vi "SDCP SMF Transmitter and Receiver - Obtain Plot Points from Trace File.vi"(4 "Stop file index":u16, 6 "error in (no error)":errorcluster, 7 "Trace File Path":path=path "E:/Projects/System Diagnostics and Control Protocol/SDCP_LabVIEW/temp/Trace Files/21 Apr 2024 20-17.csv", 8 "Start file index":u16, 10 "Parameter file path":path=path "E:/Projects/System Diagnostics and Control Protocol/SDCP_LabVIEW/Parameter Files/Motion_Processing.param") -> (0 "error out":errorcluster, 2 "Parameter names":string[](array[string]), 3 "Plot details":T1(array[cluster]))   [LabVIEW 2020]
panel:
  out "File counter":i32
  out "Frame Counter":u16
  in  "Parameter Length":i32=1
  in  "Parameter Start Index":i32=26
  out "XY Graph":T2(graph)
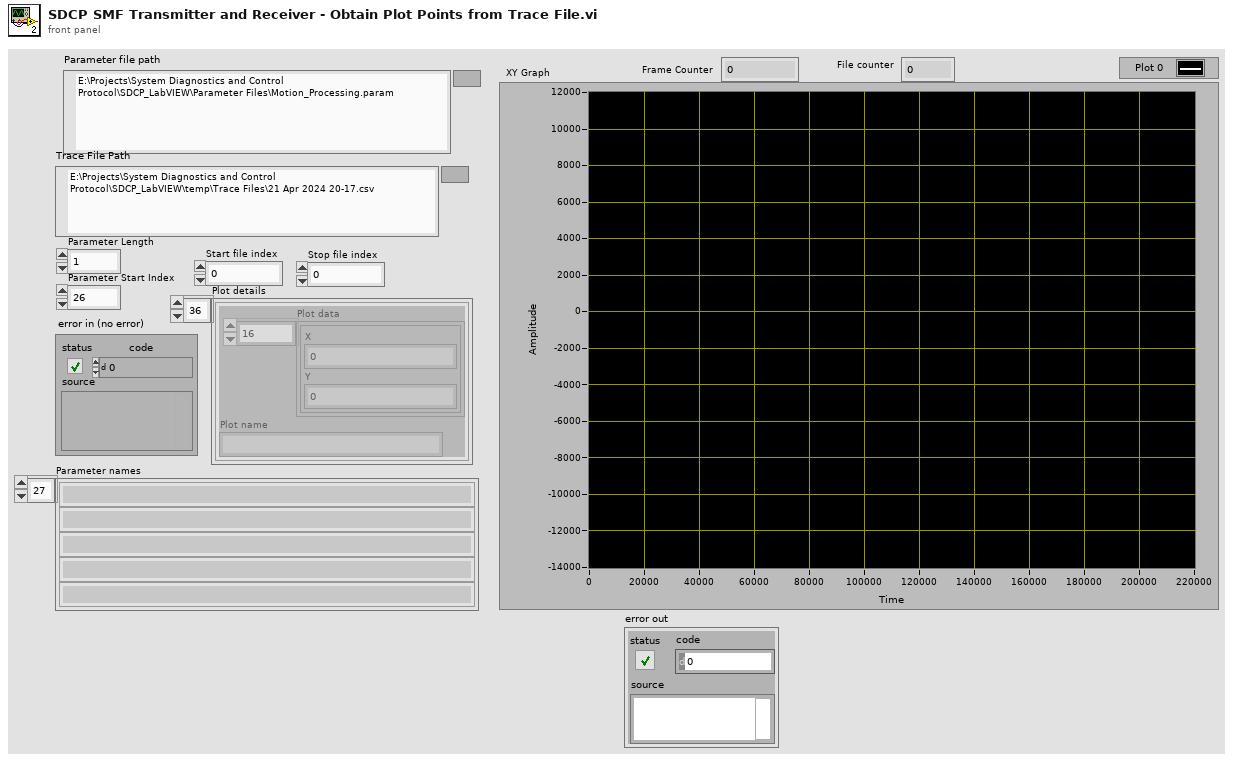
[diagram p1: front panel]
types:
  T1 = cluster{"Plot data":cluster{"X":dbl, "Y":dbl}[], "Plot name":string}[]
  T2 = cluster{"Plot data":cluster{"X":dbl, "Y":dbl}[]}[]
  T3 = cluster{"Plot data":cluster{"X":dbl, "Y":dbl}[], "Plot name":string}
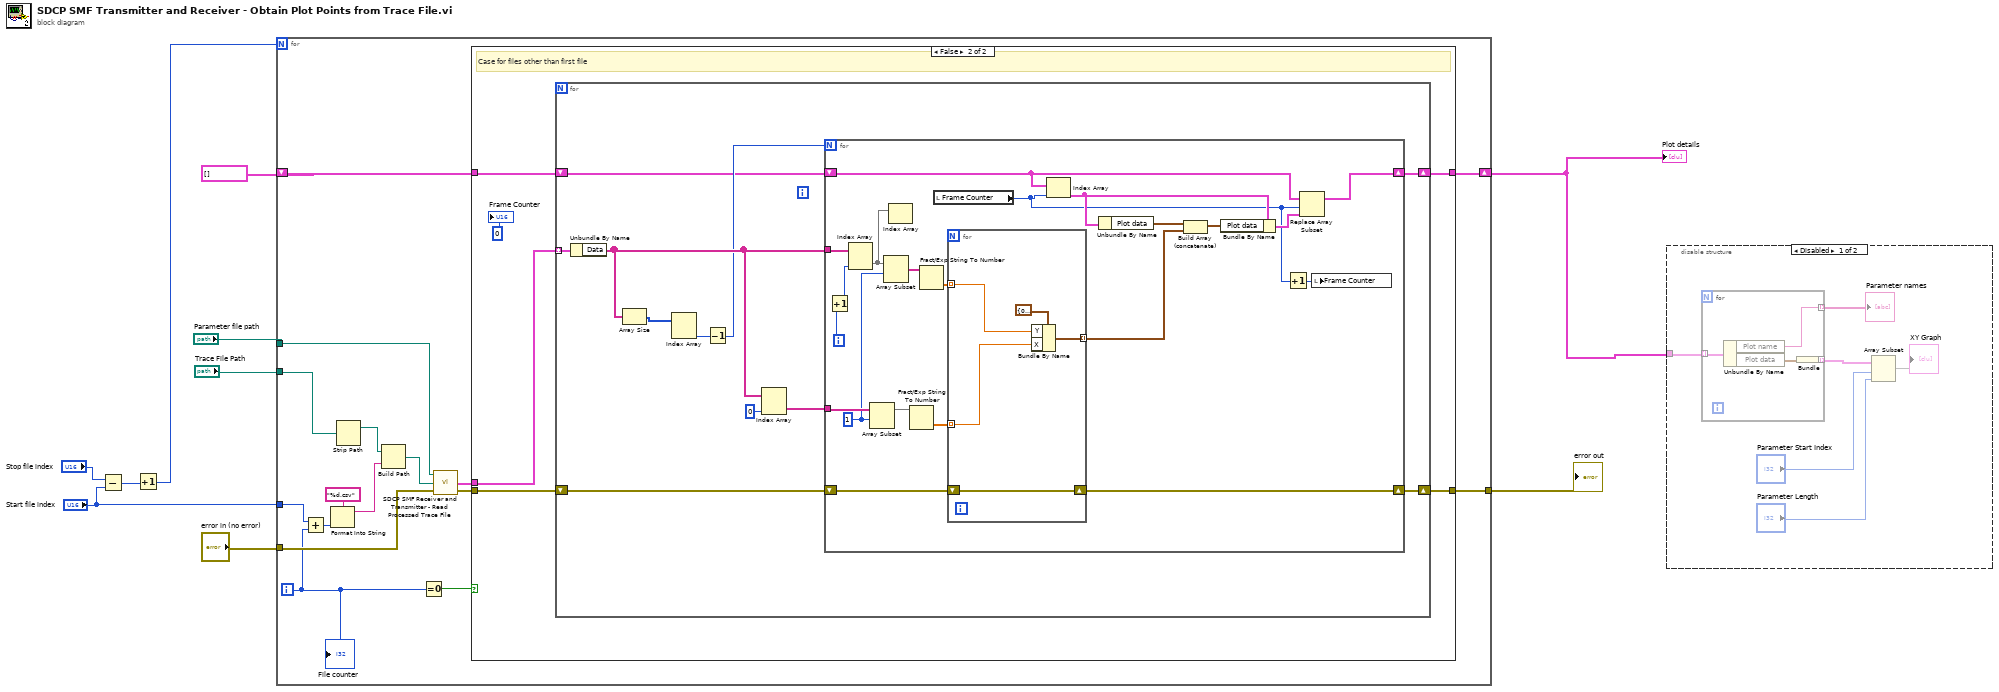
[diagram p0: block diagram]
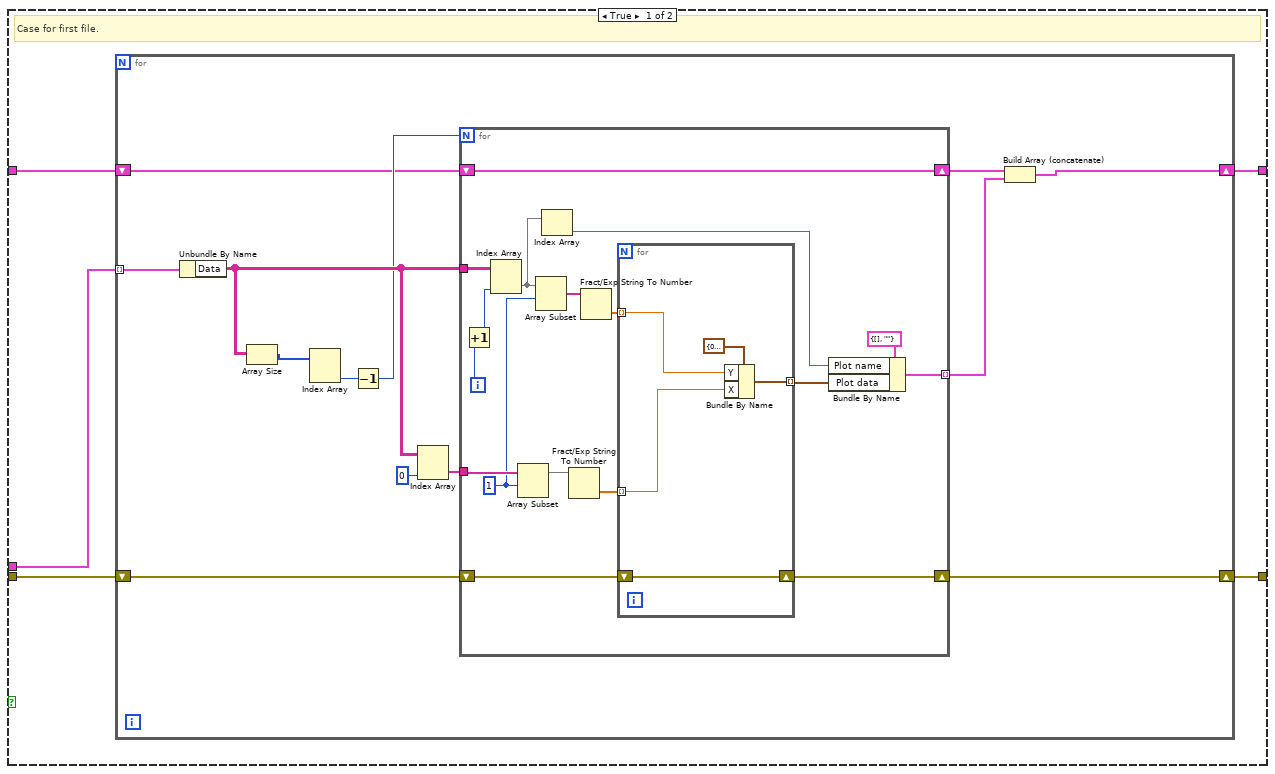
[diagram p3: hidden frame]
diagram:
  n1 = Subtract(x="Stop file index", y="Start file index") -> (x-y=w2:u16)
  n2 = Increment(x=w2) -> (x+1=w1:u16)
  n3 = for {
    N: w1 -> [_]
    tunnel: "Parameter file path" -> [w26]
    tunnel: "Trace File Path" -> [w20]
    tunnel: "error in (no error)" -> [w25]
    shift-right: [w21] -> w6
    shift-left: T1 [] -> [w22]
    tunnel: [w15] -> w5
    tunnel: "Start file index" -> [w11]
    i -> [w12]
    n4 = Add(x=w11, y=w12) -> (x+y=w13:i32)
    n5 = Format Into String(format string="%d.csv", w13) -> (resulting string=w16:string)  [unwired: 2 in, 1 out]
    n6 = Strip Path(path=w20) -> (stripped path=w19:path)  [unwired: 1 out]
    n7 = Build Path(base path=w19, name or relative path=w16) -> (appended path=w18:path)
    n8 = Equal To 0?(x=w12) -> (x = 0?=w14:bool)
    n9 = call "SDCP SMF Receiver and Transmitter - Read Processed Trace File.vi"("error in (no error)"=w25, "Trace File Path"=w18, "Parameter file path"=w26) -> ("error out"=w24:errorcluster, "Framewise output"=w23:cluster{"Data":string[][]}[])  [unwired: 1 out]
    n10 = case shown="False" w14 {
      tunnel: w24 -> [w31 w72]
      tunnel: w23 -> [w30 w71]
      tunnel: w22 -> [w29 w70]
      tunnel: [w28 w69] -> w21
      tunnel: [w27 w68] -> w15
      frame True {
        # "Case for first file."
        n11 = for {
          shift-right: [w37] -> w27
          shift-left: w31 -> [w41]
          tunnel: w30 -> [w44] mode=indexing
          shift-right: [w33] -> w28
          shift-left: w29 -> [w36]
          n12 = Unbundle By Name(w44) -> ("Data"=w40:string[][])
          n13 = Array Size(array=w40) -> (size(s)=w43:i32[])
          n14 = Index Array(array=w43) -> (element #2=w42:i32)  [unwired: 2 in, 1 out]
          n15 = Decrement(x=w42) -> (x-1=w39:i32)
          n16 = Index Array(array=w40, index (col)=0 ("disabled index (col)")) -> (element=w38:string[])  [unwired: 1 in]
          n17 = for {
            N: w39 -> [_]
            shift-right: [w46] -> w37
            shift-left: w41 -> [w47]
            tunnel: w40 -> [w61]
            tunnel: w38 -> [w55]
            tunnel: [w49] -> w34 mode=indexing
            shift-right: [w48] -> w35
            shift-left: w36 -> [w48]
            i -> [w60]
            w52 = 1 ("index")
            n18 = Increment(x=w60) -> (x+1=w45:i32)
            n19 = Index Array(array=w61, index (col)=w45) -> (element=w51:string[])  [unwired: 1 in]
            n20 = Array Subset(array=w55, index=w52) -> (w54:string[])  [unwired: 1 in]
            n21 = Array Subset(array=w51, index=w52) -> (w53:string[])  [unwired: 1 in]
            n22 = Index Array(array=w51) -> (element=w50:string)  [unwired: 1 in]
            n23 = Fract/Exp String To Number(string=w54) -> (number=w58:dbl[])  [unwired: 3 in, 1 out]
            n24 = Fract/Exp String To Number(string=w53) -> (number=w59:dbl[])  [unwired: 3 in, 1 out]
            n25 = for {
              tunnel: w59 -> [w64] mode=indexing
              tunnel: w58 -> [w65] mode=indexing
              tunnel: [w63] -> w56 mode=indexing
              shift-right: [w62] -> w46
              shift-left: w47 -> [w62]
              n26 = Bundle By Name(cluster=cluster{"X":dbl, "Y":dbl} {"X"=0.0, "Y"=0.0}, "Y"=w64, "X"=w65) -> (w63:cluster{"X":dbl, "Y":dbl})
            }
            n27 = Bundle By Name(cluster=T3 {"Plot data"=[], "Plot name"=""}, "Plot name"=w50, "Plot data"=w56) -> (w49:T3)
          }
          n28 = Build Array (concatenate)(w35, w34) -> (w33:T1)
        }
      }
      frame False {
        # "Case for files other than first file"
        n29 = for {
          shift-right: [w76] -> w68
          shift-left: w72 -> [w80]
          tunnel: w71 -> [w83] mode=indexing
          shift-right: [w74] -> w69
          shift-left: w70 -> [w75]
          n30 = Unbundle By Name(w83) -> ("Data"=w79:string[][])
          n31 = Array Size(array=w79) -> (size(s)=w82:i32[])
          n32 = Index Array(array=w82) -> (element #2=w81:i32)  [unwired: 2 in, 1 out]
          n33 = Decrement(x=w81) -> (x-1=w78:i32)
          n34 = Index Array(array=w79, index (col)=0 ("disabled index (col)")) -> (element=w77:string[])  [unwired: 1 in]
          n35 = for {
            N: w78 -> [_]
            shift-right: [w94] -> w76
            shift-left: w80 -> [w95]
            tunnel: w79 -> [w104]
            tunnel: w77 -> [w100]
            shift-right: [w86] -> w74
            shift-left: w75 -> [w88]
            i -> [w103]
            w97 = 1 ("index")
            n36 = Increment(x=w103) -> (x+1=w93:i32)
            n37 = Index Array(array=w104, index (col)=w93) -> (element=w96:string[])  [unwired: 1 in]
            n38 = Array Subset(array=w100, index=w97) -> (w99:string[])  [unwired: 1 in]
            n39 = Array Subset(array=w96, index=w97) -> (w98:string[])  [unwired: 1 in]
            n40 = Index Array(array=w96) -> ()  [unwired: 1 in, 1 out]
            n41 = Fract/Exp String To Number(string=w99) -> (number=w101:dbl[])  [unwired: 3 in, 1 out]
            n42 = Fract/Exp String To Number(string=w98) -> (number=w102:dbl[])  [unwired: 3 in, 1 out]
            n43 = local read "Frame Counter"() -> (w85:u16)
            n44 = for {
              tunnel: w102 -> [w107] mode=indexing
              tunnel: w101 -> [w108] mode=indexing
              tunnel: [w106] -> w92 mode=indexing
              shift-right: [w105] -> w94
              shift-left: w95 -> [w105]
              n45 = Bundle By Name(cluster=cluster{"X":dbl, "Y":dbl} {"X"=0.0, "Y"=0.0}, "Y"=w107, "X"=w108) -> (w106:cluster{"X":dbl, "Y":dbl})
            }
            n46 = Index Array(array=w88, index=w85) -> (element=w90:T3)
            n47 = Unbundle By Name(w90) -> ("Plot data"=w91:cluster{"X":dbl, "Y":dbl}[])
            n48 = Build Array (concatenate)(w91, w92) -> (w89:cluster{"X":dbl, "Y":dbl}[])
            n49 = Bundle By Name(cluster=w90, "Plot data"=w89) -> (w87:T3)
            n50 = Increment(x=w85) -> (x+1=w84:u16)
            n51 = Replace Array Subset(array=w88, new element=w87, index=w85) -> (w86:T1)
            n52 = local write "Frame Counter"(w84) -> ()
          }
        }
        "Frame Counter" <- u16 0 ("Frame Counter")
      }
    }
    "File counter" <- w12
  }
  "Plot details" <- w6
  "error out" <- w5
  n53 = disable-structure shown="Disabled" {
    disable-tunnel: w6 -> [w110 _]
    frame Disabled {
      n54 = for {
        tunnel: w110 -> [w119] mode=indexing
        tunnel: [w117] -> w114 mode=indexing
        tunnel: [w116] -> w115 mode=indexing
        n55 = Unbundle By Name(w119) -> ("Plot name"=w116:string, "Plot data"=w118:cluster{"X":dbl, "Y":dbl}[])
        n56 = Bundle("Plot data"=w118) -> (w117:cluster{"Plot data":cluster{"X":dbl, "Y":dbl}[]})  [unwired: 1 in]
      }
      "Parameter names" <- w115
      n57 = Array Subset(array=w114, index="Parameter Start Index", length="Parameter Length") -> (→"XY Graph":T2)
    }
    frame Enabled {
    }
  }
